vi "日志存储 (子VI).vi"(11 "data in":T1) -> ()   [LabVIEW 2016, in "MB SLAVE.lvlib"]
uses:
  MB SLAVE.lvlib
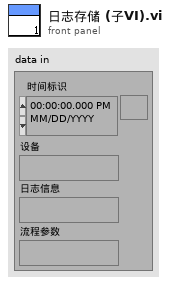
[diagram p1: front panel]
types:
  T1 = cluster{"时间标识":timestamp, "设备":string, "日志信息":string, "流程参数":string}
  T2 = typedef "数据库类型.ctl" = enum16{"Access", "SQLite"}
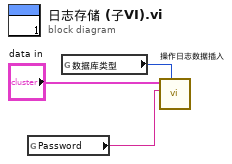
[diagram p0: block diagram]
diagram:
  n1 = global read "modbus slave全局.vi" "Password"() -> (w1:string)
  n2 = global read "modbus slave全局.vi" "数据库类型"() -> (w3:T2)
  n3 = call "操作日志数据插入.vi"("data"="data in", "Password"=w1, "数据库类型"=w3) -> ()  [unwired: 7 in, 1 out]
